vi "veristandSteps-installer-updateVeriStandProgramFilesPath.vi"(8 "error in (no error)":errorcluster, 10 "VeriStand Applicatin Program Files Directroy":string, 11 "InstallerMutationSession":T1={"Installer Build Specification Ref"=refnum, "Project reference out"=refnum, "Installer Project Path"=path "C:/Users/Public/Documents/Git-Source/VeriStand-Custom-Steps-For-TestStand/Source/LabVIEW Code/Installer/Installer - Copy.lvproj"}) -> (0 "error out":errorcluster, 3 "InstallerMutationSession out":T1={"Installer Build Specification Ref"=refnum, "Project reference out"=refnum, "Installer Project Path"=path "C:/Users/Public/Documents/Git-Source/VeriStand-Custom-Steps-For-TestStand/Source/LabVIEW Code/Installer/Installer - Copy.lvproj"})   [LabVIEW 2014, in "veristand-steps-build-system.lvlib"]
uses:
  veristand-steps-build-system.lvlib
  lv-build-system/types/LVInstallerMutationSession.ctl
  lv-build-system/lv-build-library.lvlib
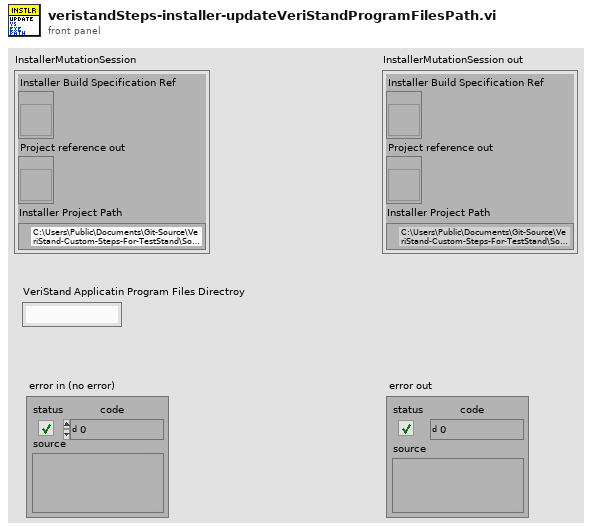
[diagram p1: front panel]
types:
  T1 = typedef "lv-build-library.lvlib/LVInstallerMutationSession.ctl" = cluster{"Installer Build Specification Ref":refnum<vi>, "Project reference out":refnum<vi>, "Installer Project Path":path}
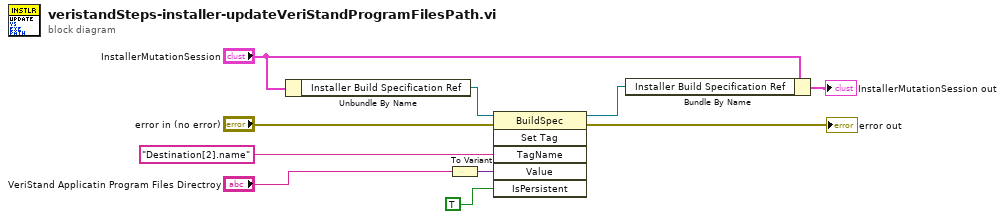
[diagram p0: block diagram]
diagram:
  n1 = Unbundle By Name("InstallerMutationSession") -> ("Installer Build Specification Ref"=w4:refnum<vi>)
  n2 = To Variant(anything="VeriStand Applicatin Program Files Directroy") -> (Variant=w7:variant)
  n3 = invoke class="BuildSpec" method="Set Tag"(reference=w4, error in="error in (no error)", "TagName"="Destination[2].name" ("Tag Name"), "Value"=w7, "IsPersistent"=TRUE ("Is Persistent")) -> (reference out=w2:refnum<vi>, error out=→"error out":errorcluster)  [unwired: 1 in, 4 out]
  n4 = Bundle By Name(cluster="InstallerMutationSession", "Installer Build Specification Ref"=w2) -> (→"InstallerMutationSession out":T1)
